vi "JX_ConvertNumToReg.vi"(10 "Steps":sgl, 11 "Direction":bool) -> (3 "Array":u16[](array[numeric]))   [LabVIEW 2023, in "Jiaxin_Stepper_Controller.lvlib"]
uses:
  Jiaxin_Stepper_Controller.lvlib
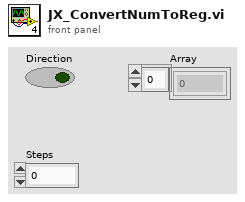
[diagram p1: front panel]
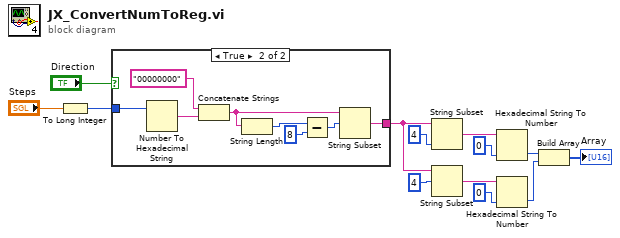
[diagram p0: block diagram]
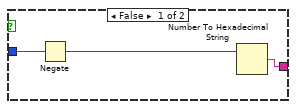
[diagram p2: hidden frame]
diagram:
  n1 = To Long Integer(number="Steps") -> (32bit integer=w12:i32)
  n2 = case shown="True" "Direction" {
    tunnel: [w14 w19] -> w11
    tunnel: w12 -> [w15 w18]
    frame False {
      n3 = Negate(x=w15) -> (-x=w16:i32)
      n4 = Number To Hexadecimal String(2:w16) -> (0:w14:string)  [unwired: 1 in]
    }
    frame True {
      n5 = Number To Hexadecimal String(2:w18) -> (0:w17:string)  [unwired: 1 in]
      n6 = Concatenate Strings("00000000", w17) -> (w24:string)
      n7 = String Length(string=w24) -> (length=w23:i32)
      n8 = Subtract(x=w23, y=8) -> (x-y=w21:i32)
      n9 = String Subset(string=w24, offset (0)=w21) -> (substring=w19:string)  [unwired: 1 in]
    }
  }
  n10 = String Subset(string=w11, length (rest)=4 ("length (rest)")) -> (substring=w7:string)  [unwired: 1 in]
  n11 = String Subset(string=w11, offset (0)=4) -> (substring=w5:string)  [unwired: 1 in]
  n12 = Hexadecimal String To Number(string=w7, default (0uL)=u16 0 ("default (0 U32)")) -> (number=w3:u16)  [unwired: 1 in, 1 out]
  n13 = Hexadecimal String To Number(string=w5, default (0uL)=u16 0 ("default (0 U32)")) -> (number=w2:u16)  [unwired: 1 in, 1 out]
  n14 = Build Array(w3, w2) -> (→"Array":u16[])
